vi "GetHostname.vi"(8 "error in (no error)":errorcluster) -> (0 "error out":errorcluster, 3 "hostname":string)   [LabVIEW 2017, in "SystemInfoProcess.lvlib"]
doc: "Gets the system hostname."
uses:
  <vilib>/addons/SystemInfoProcess/SystemInfoProcess.lvlib
  <vilib>/addons/PointValueMap/subVIs/Point_Read_string.vi
  <vilib>/addons/PointValueMap/PointValueMap.lvlib
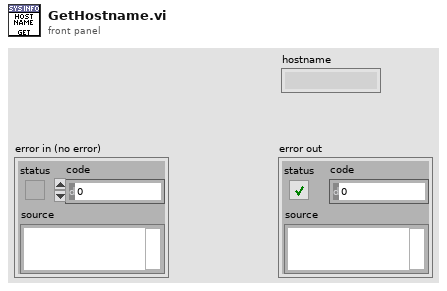
[diagram p1: front panel]
types:
  T1 = typedef "PointValueMap.lvlib/PointMap.ctl" = refnum<data-value>
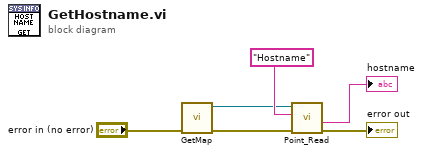
[diagram p0: block diagram]
diagram:
  n1 = call <vilib>:"GetMap.vi"("error in (no error)"="error in (no error)") -> ("error out"=w3:errorcluster, "SystemInfoMap"=w2:T1)  [unwired: 9 in]
  n2 = call-poly <vilib>:"Point_Read.vi"("Error In"=w3, "Tag"="Hostname", "Map"=w2) -> ("Error Out"=→"error out":errorcluster, "Value"=→"hostname":string)  [unwired: 3 in, 4 out]
